vi "ROI entry screen-main buttons management.vi"(6 "Imaging button boolean text":string=". . .", 7 "Acquisition button boolean text":string=". . .", 8 "Imaging button disabled?":T1(ring), 9 "Acquisition button disabled?":T1(ring), 10 "Done button disabled?":T1(ring)) -> ()   [LabVIEW 2013]
uses:
  Globals/gl_ROI Entry UI globals.vi
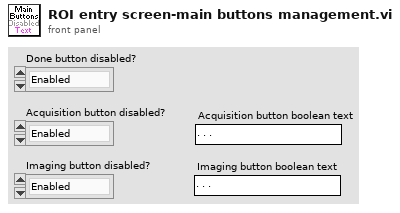
[diagram p1: front panel]
types:
  T1 = enum8{"Enabled", "Disabled", "Disabled and Grayed Out"}
  T2 = typedef "ROI entry screen ctrl refs cluster.ctl" = cluster{"Done button":refnum<vi>, "Imaging button":refnum<vi>, "Acquisition button":refnum<vi>, "POI dwell time (us)":refnum<vi>, "Scan dwell time per pixel (us)":refnum<vi>, "# of planes":refnum<vi>, "Zoom":refnum<vi>, "Equal size":refnum<vi>, "Channel":refnum<vi>, "Image Display":refnum<vi>, "Z-Plane Selector":refnum<vi>, "Number of lines left":refnum<vi>, "Z-stack folder path":refnum<vi>, "POI Density":refnum<vi>, "Arb Plane Entry":refnum<vi>, "Whole plane":refnum<vi>, "Clear Last":refnum<vi>, "Clear All":refnum<vi>, "Trial Length (sec)":refnum<vi>, "Palette Type":refnum<vi>, "Intensity slider":refnum<vi>, "# POI":refnum<vi>, "Max Z Proj":refnum<vi>, "Zplane ind":refnum<vi>, "Wavelength (nm)":refnum<vi>, "Number of Trials":refnum<vi>, "Funct stim.trig.enable":refnum<vi>, "Funct stim.trig.delay (s)":refnum<vi>, "Line Mode":refnum<vi>, "Step size (µm)":refnum<vi>, "ROI move mode":refnum<vi>, "Cool-down time (s)":refnum<vi>, "Enable cool-down time":refnum<vi>, "Motor Z ind. (um)":refnum<vi>, "AOL Z ind. (um)":refnum<vi>}
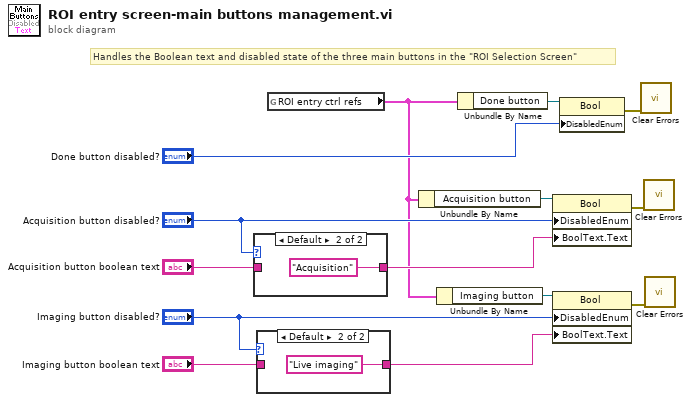
[diagram p0: block diagram]
diagram:
  # "Handles the Boolean text and disabled state of the three main buttons in the \"ROI Selection Screen\""
  n1 = case shown="Default" "Acquisition button disabled?" {
    tunnel: [w15 "Acquisition" ("Boolean Text.Text")] -> w5
    tunnel: "Acquisition button boolean text" -> [w15 _]
    frame "Enabled" {
    }
    frame Default {
    }
  }
  n2 = case shown="Default" "Imaging button disabled?" {
    tunnel: [w17 "Live imaging" ("Boolean Text.Text")] -> w11
    tunnel: "Imaging button boolean text" -> [w17 _]
    frame "Enabled" {
    }
    frame Default {
    }
  }
  n3 = global read "gl_ROI Entry UI globals.vi" "ROI entry ctrl refs"() -> (w4:T2)
  n4 = Unbundle By Name(w4) -> ("Acquisition button"=w9:refnum<vi>)
  n5 = Unbundle By Name(w4) -> ("Imaging button"=w10:refnum<vi>)
  n6 = Unbundle By Name(w4) -> ("Done button"=w14:refnum<vi>)
  n7 = property on="Property Node" class="Bool"(reference=w9, "DisabledEnum"="Acquisition button disabled?", "BoolText.Text"=w5) -> (error out=w1:errorcluster)  [unwired: 1 in, 1 out]
  n8 = property on="Property Node" class="Bool"(reference=w10, "DisabledEnum"="Imaging button disabled?", "BoolText.Text"=w11) -> (error out=w2:errorcluster)  [unwired: 1 in, 1 out]
  n9 = property on="Property Node" class="Bool"(reference=w14, "DisabledEnum"="Done button disabled?") -> (error out=w3:errorcluster)  [unwired: 1 in, 1 out]
  n10 = call <vilib>:"Clear Errors.vi"("error in (no error)"=w3) -> ()  [unwired: 6 in, 1 out]
  n11 = call <vilib>:"Clear Errors.vi"("error in (no error)"=w1) -> ()  [unwired: 6 in, 1 out]
  n12 = call <vilib>:"Clear Errors.vi"("error in (no error)"=w2) -> ()  [unwired: 6 in, 1 out]
